vi "play-AFM-CS-imaging.vi"() -> ()   [LabVIEW 2017]
uses:
  z-axis-params.ctl
  <vilib>/userdefined/High Color/nirio_resource_hc.ctl
  controls/expMetaData.ctl
  <vilib>/Utility/file.llb/Read Delimited Spreadsheet (DBL).vi
  <vilib>/FPGAPlugInAG/cRIO-9082/niLvFpga_Open_cRIO-9082.vi
  <vilib>/rvi/interface/common/dynamic/niFpgaDynamicAddResources.vi
  <vilib>/FPGAPlugInAG/Dynamic/niLvFpga_Reset_Dynamic.vi
  <vilib>/rvi/interface/common/niFpgaWaitOnOcc.vi
  <vilib>/Utility/error.llb/Error Cluster From Error Code.vi
  <vilib>/rvi/errors/niLvFpgaAdjustHostInterfaceError.vi
  <vilib>/FPGAPlugInAG/Dynamic/niLvFpga_Run_Dynamic.vi
  <vilib>/Utility/file.llb/Write Delimited Spreadsheet (DBL).vi
  <vilib>/FPGAPlugInAG/Dynamic/niLvFpga_Close_Dynamic.vi
  <userlib>/_matio/level5/Public/Write/Append Data Element.llb/Append Data Element (Anything).vi
  <vilib>/rvi/interface/nirviOpenFPGA/nirviOpenFPGA.xnode
  FPGA Bitfiles/afmimagingcontro_FPGATargetSPARTA_cs-scanning_gCu814jKz54.lvbitx
  <vilib>/rvi/interface/nirviMethod/nirviMethod.xnode
  <vilib>/rvi/interface/nirviReadWriteControl/nirviReadWriteControl.xnode
  <vilib>/rvi/interface/nirviCloseFPGA/nirviCloseFPGA.xnode
  <vilib>/FPGAPlugInAG/Dynamic/niLvFpga_ConfigureFifo_Dynamic.vi
  <vilib>/rvi/errors/niLvFpgaMergeErrorWithErrorCode.vi
  <vilib>/rvi/interface/Simulation/niFpgaSimulationCallBeginRW.vi
  <vilib>/FPGAPlugInAG/Dynamic/niLvFpga_ReadFifo_Dynamic.vi
  NiFpgaLv.dll
  <userlib>/_matio/level5.lvlib
  <vilib>/FPGAPlugInAG/Dynamic/niLvFpga_WriteFifo_Dynamic.vi
panel:
  out "Current Case":i16
  out "state counts":u64[](array[numeric])
  out "iter":i32
  out "entity-index":i16
  out "x = 0?":bool
  out "Numeric":i32
  out "error out 2":errorcluster
  out "boolean  indicators":T1
  in  "Tab Control":T2(tab)
  in  "init Z up":sgl step=0.5
  in  "trigger-0":bool
  in  "numEntities":i16
  in  "data-root":path=path "C:/Users/arnold/Documents/labview/afm_imaging/data"
  in  "TsTicks":u32=1600
  in  "collect all":bool
  in  "collect move":bool
  in  "Ki-xy":sgl=0.005
  in  "z-axis-params":T3={"TOL"=0.3, "ramp_rate"=-5e-05, "z_u_max"=5.0, "setpoint"=0.0, "Ki"=0.01, "Z_error_threshold"=0.05, "Z_settled_samples_threshold "=500, "z_UP"=1.5, "zup_N"=500} {"Z_error_threshold" format="%#_13g"; "ramp_rate" format="%#_4g"; "TOL" format="%#_13g"}
  in  "step_down_frac":fxp<+,8,1>=1.0
  in  "input-file-name":string="cs-traj10-500.csv"
  out "output-data-path":path
  out "output-meta-data-path":path
  in  "note-blob":string
  in  "overwrite":bool
  in  "xy settled-samples\n threshold":i16=200
  in  "xy error-threshold":sgl=0.1
  out "number-settled-samples-x":i16
  out "number-settled-samples-y":i16
  out "case-selected":i16
  out "e(0) (threshhold init)":fxp<+/-,16,5>
  out "size(s)":i32
  out "nsamps":i32
  out "elements left":i32=1
  out "y iter":i32
  out "size(s) 2":i32[](array[numeric])
  out "Array":i32[][](array[numeric])
  out "z-control":dbl[](graph)
  out "x-axis":dbl[](graph)
  out "z-error":dbl[](graph)
  out "y-axis":dbl[](graph)
  in  "STOP":bool
  # "- If collect all = fasle and collect move = false,\nwe only collect measurement data.\n- If collect all = false, and collect move = true,\nwe collect measurement and move data.\n- If collect all = true, we collect everything."
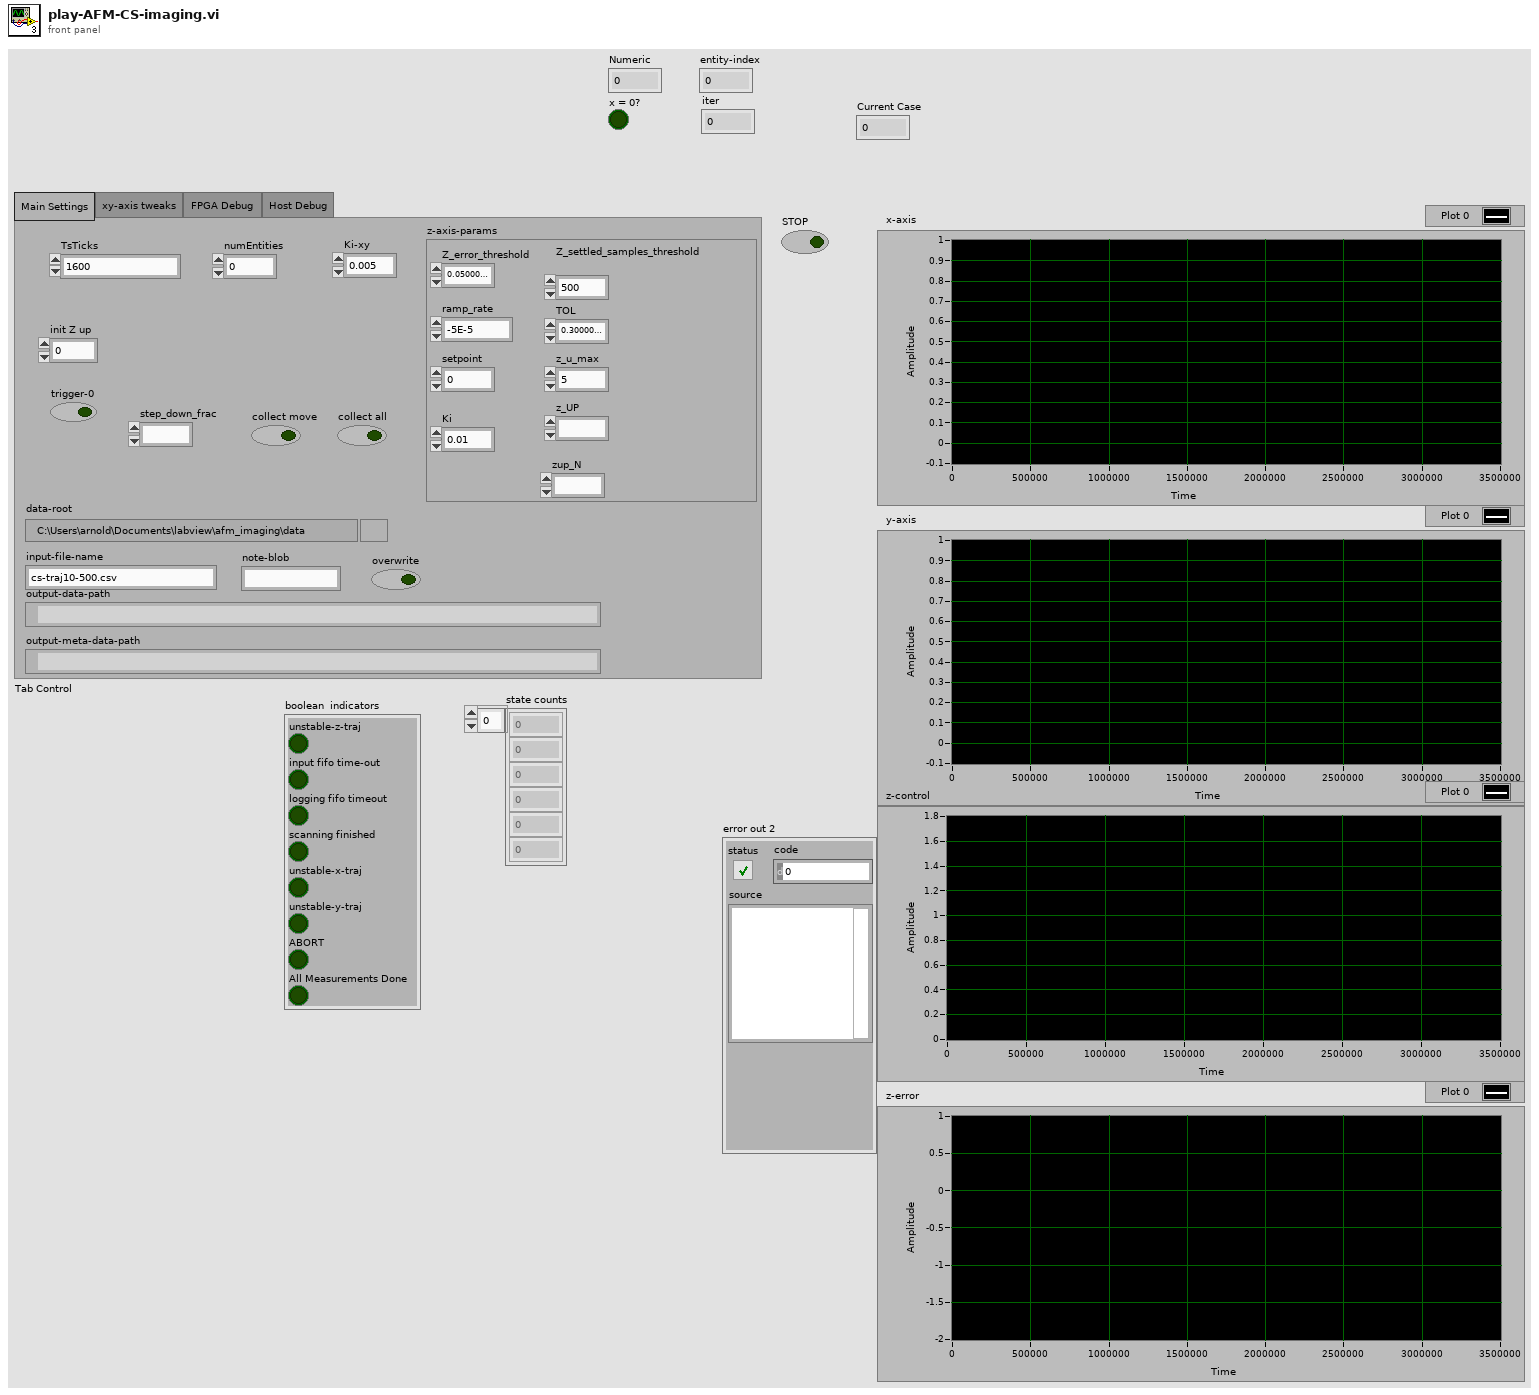
[diagram p1: front panel]
types:
  T1 = cluster{"unstable-z-traj":bool, "input fifo time-out":bool, "logging fifo timeout":bool, "scanning finished":bool, "unstable-x-traj":bool, "unstable-y-traj":bool, "ABORT":bool, "All Measurements Done":bool}
  T2 = enum32{"Main Settings", "xy-axis tweaks", "FPGA Debug ", "Host Debug"}
  T3 = typedef "z-axis-params.ctl" = cluster{"TOL":sgl, "ramp_rate":sgl, "z_u_max":sgl, "setpoint":sgl, "Ki":sgl, "Z_error_threshold":sgl, "Z_settled_samples_threshold ":i16, "z_UP":fxp<+/-,16,5>, "zup_N":i16}
  T4 = typedef "nirio_resource_hc.ctl" = tag
  T5 = enum16{"open", "replace", "create", "open or create", "replace or create", "replace or create with confirmation"}
  T6 = typedef "expMetaData.ctl" = cluster{"xy_error_threshold":sgl, "xy_settled_samples_threshold":i16, "Ki_xy":sgl, "state_counts":dbl[], "TOL":sgl, "ramp_rate":sgl, "z_u_max":sgl, "setpoint":sgl, "Ki":sgl, "Z_error_threshold":sgl, "Z_settled_samples_threshold ":i16, "z_UP":sgl, "zup_N":i16}
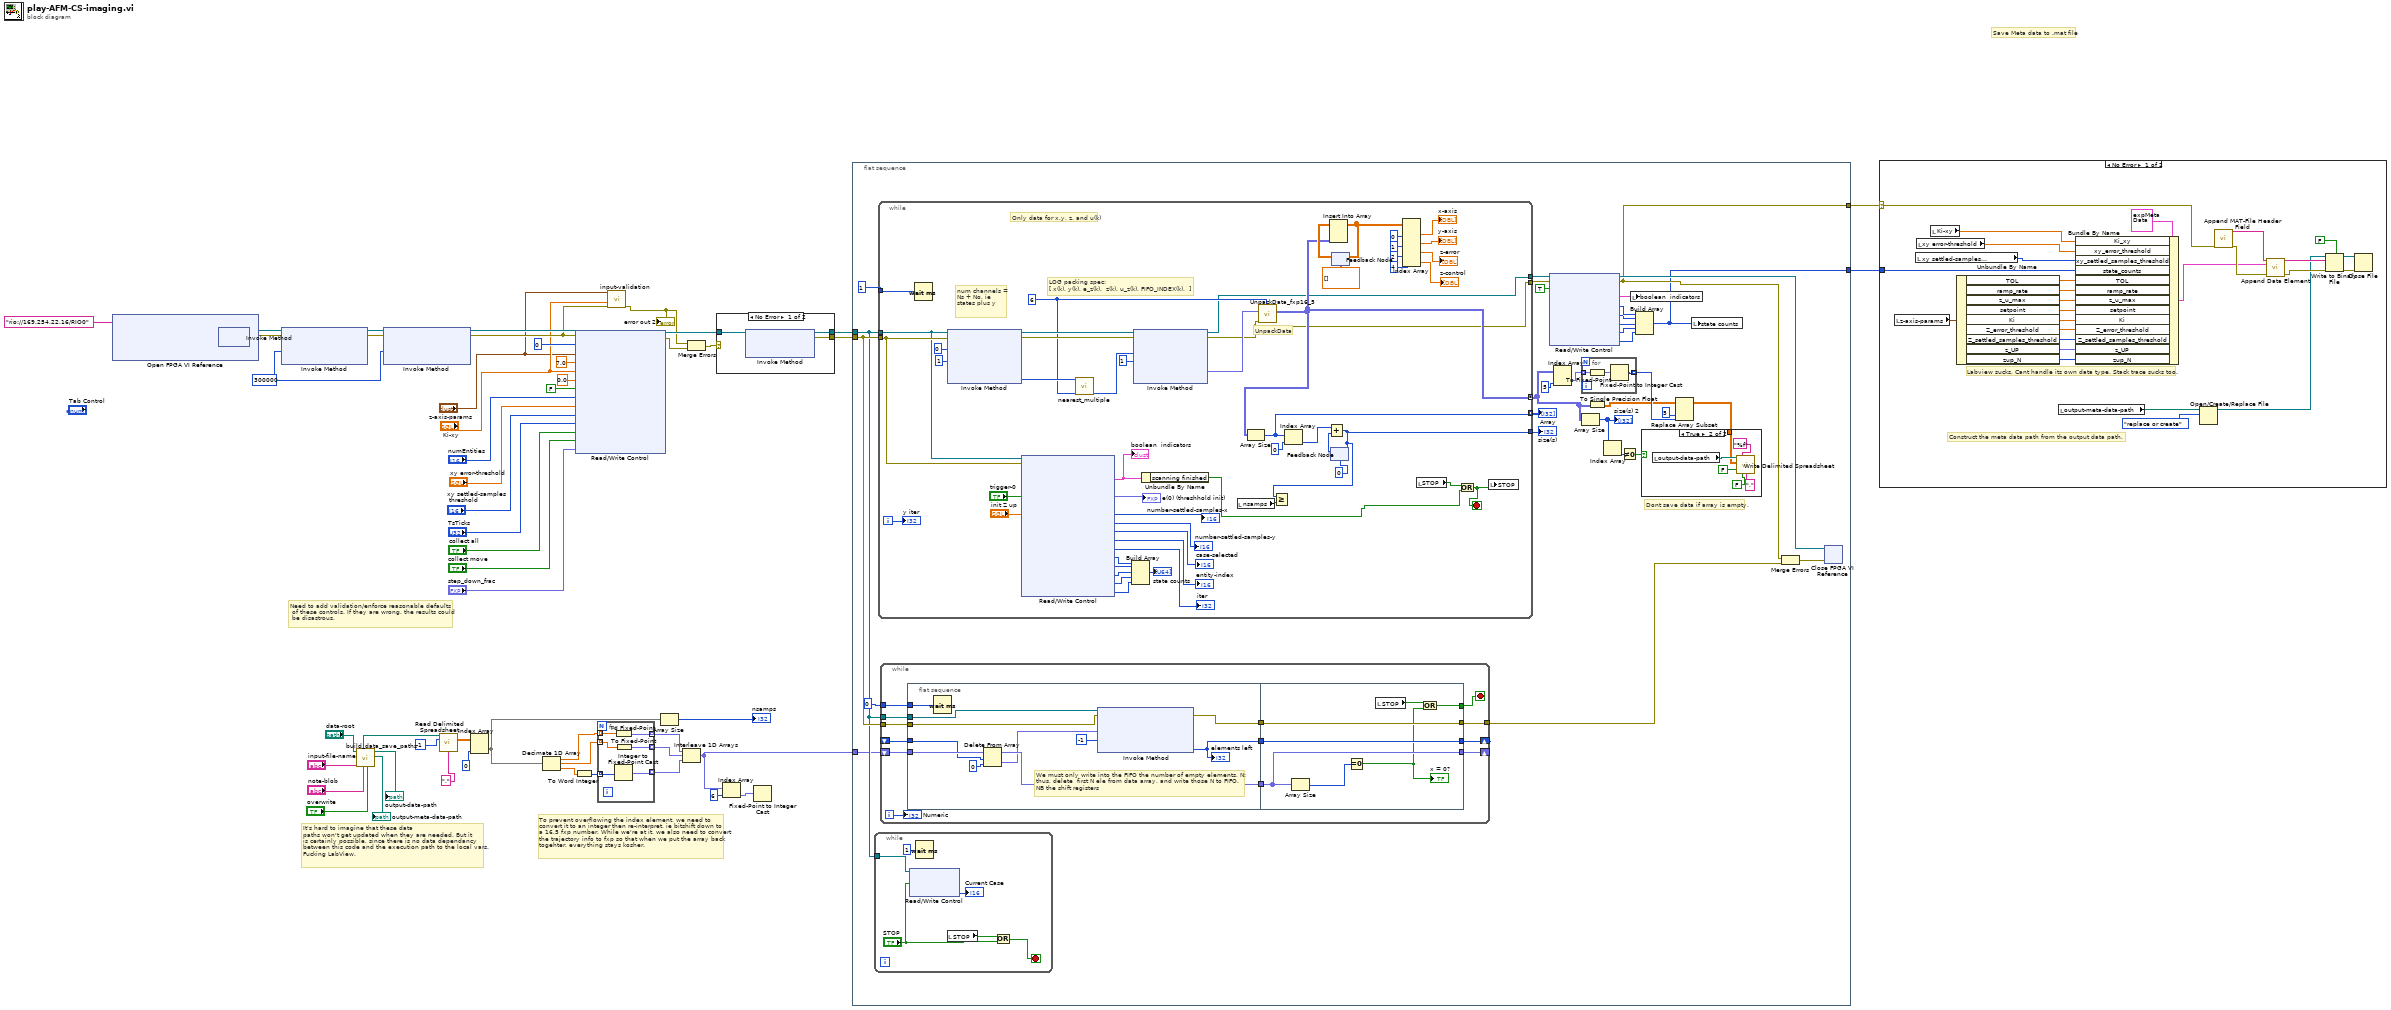
[diagram p0: block diagram]
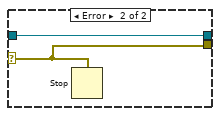
[diagram p4: hidden frame]
diagram:
  w53 = 300000
  # "It's hard to imagine that these data\npaths won't get updated when they are needed. But it \nis certainly possible, since there is no data dependancy \nbetween this code and the execution path to the local vars.\nFucking LabView."
  # "Save Meta data to .mat file"
  # "To prevent overflowing the index element, we need to \nconvert it to an integer then re-interpret, ie bitshift down to \na 16,5 fxp number. While we're at it, we also need to convert\nthe trajectory info to fxp so that when we put the array back\ntogehter, everything stays kosher."
  # "Need to add validation/enforce reasonable defaults\n of these controls. If they are wrong, the results could\n be disastrous."
  n1 = xnode "Open FPGA VI Reference"("resource name"=T4 "rio://169.254.22.16/RIO0") -> ("FPGA VI Reference Out"=w52:refnum<k20>, "error out"=w51:errorcluster)  [unwired: 1 in]
  n2 = xnode "Invoke Method"("FPGA VI Reference In"=w52, "error in"=w51) -> ("FPGA VI Reference Out"=w44:refnum<k20>, "error out"=w43:errorcluster)
  n3 = xnode "Invoke Method"("FPGA VI Reference In"=w44, "error in"=w43, "Requested Depth"=w53) -> ("FPGA VI Reference Out"=w46:refnum<k20>, "error out"=w47:errorcluster)  [unwired: 1 out]
  n4 = call "build_data_save_paths.vi"("overwrite"="overwrite", "note-blob"="note-blob", "base-file-name"="input-file-name", "data-root"="data-root") -> ("output-meta-data-path"=→"output-meta-data-path":path, "output-data-path"=→"output-data-path":path, "input-data-path"=w3:path)  [unwired: 3 in, 2 out]
  n5 = xnode "Invoke Method"("FPGA VI Reference In"=w46, "error in"=w47, "Requested Depth"=w53) -> ("FPGA VI Reference Out"=w54:refnum<k20>, "error out"=w29:errorcluster)  [unwired: 1 out]
  n6 = call-poly <vilib>:"Read Delimited Spreadsheet.vi"("file path (dialog if empty)"=w3, "number of rows (all:-1)"=-1, "delimiter (\\t)"=",") -> ("all rows"=w38:dbl[][])  [unwired: 7 in, 5 out]
  n7 = Index Array(array=w38, index (col)=0 ("dimension size")) -> (element=w14:dbl[])  [unwired: 1 in]
  n8 = Decimate 1D Array(w14) -> (w22:dbl[], w21:dbl[], w23:dbl[])
  n9 = xnode "Read/Write Control"("FPGA VI Reference In"=w54, "error in"=w29, "initial case"=i16 0, "z-axis-params"="z-axis-params", "xy-bound"=sgl 7.0, "Ki-xy"="Ki-xy", "init Z up"=sgl 0.0 ("u(0)"), "trigger-0"=FALSE, "numEntities"="numEntities", "error-threshold"="xy error-threshold", "settled-samples threshold"="xy settled-samples\n threshold", "TsTicks"="TsTicks", "collect all"="collect all", "collect move"="collect move", "step_down_frac"="step_down_frac") -> ("FPGA VI Reference Out"=w45:refnum<k20>, "error out"=w26:errorcluster)
  n10 = To Word Integer(number=w23) -> (16bit integer=w20:i16[])
  n11 = for {
    tunnel: w22 -> [w60] mode=indexing
    tunnel: w21 -> [w59] mode=indexing
    tunnel: [w58] -> w18 mode=indexing
    tunnel: [w57] -> w19 mode=indexing
    tunnel: w20 -> [w56] mode=indexing
    tunnel: [w55] -> w17 mode=indexing
    n12 = Integer to Fixed-Point Cast(integer=w56) -> (fixed-point=w55:fxp<+/-,16,5>)  [unwired: 1 in]
    n13 = To Fixed-Point(number=w60) -> (fixed-point=w57:fxp<+/-,16,5>)  [unwired: 1 in]
    n14 = To Fixed-Point(number=w59) -> (fixed-point=w58:fxp<+/-,16,5>)  [unwired: 1 in]
  }
  n15 = call "input-validation.vi"("error constant"=w29, "Ki-xy"="Ki-xy", "z-axis-params"="z-axis-params") -> ("error out"=w25:errorcluster)  [unwired: 8 in]
  "error out 2" <- w25
  n16 = Array Size(array=w14) -> (size(s)=→"nsamps":i32)
  n17 = Interleave 1D Arrays(w19, w18, w17) -> (w13:fxp<+/-,16,5>[])
  n18 = Merge Errors(w25, w26) -> (w24:errorcluster)
  n19 = case shown="No Error" w24 {
    selector: w24 -> [_ w64]
    tunnel: [w63 w64] -> w48
    tunnel: w45 -> [w62 w65]
    tunnel: [w61 w65] -> w36
    frame No Error {
      n20 = xnode "Invoke Method"("FPGA VI Reference In"=w62) -> ("FPGA VI Reference Out"=w61:refnum<k20>, "error out"=w63:errorcluster)  [unwired: 2 in]
    }
    frame Error {
      n21 = Stop(stop? (T)=w64) -> ()
    }
  }
  n22 = Index Array(array=w13, index=6) -> (element=w16:fxp<+/-,16,5>)
  n23 = Fixed-Point to Integer Cast(1:w16) -> ()  [unwired: 1 out]
  n24 = flat-sequence {
    tunnel: w48 -> [w92]
    tunnel: w36 -> [w86]
    tunnel: w13 -> [w83]
    tunnel: [w71] -> w10
    tunnel: [w70] -> w9
    frame #0 {
      # "Dont save data if array is empty."
      n25 = while {
        tunnel: w86 -> [w111]
        stop <- w107 stop-if-true
        n26 = xnode "Read/Write Control"("FPGA VI Reference In"=w111, "ABORT"="STOP") -> ("Current Case"=→"Current Case":i16)  [unwired: 1 in, 2 out]
        n27 = Wait (ms)(milliseconds to wait=u32 1) -> ()  [unwired: 1 out]
        n28 = local read "STOP"() -> (w108:bool)
        n29 = Or(x=w108, y="STOP") -> (x .or. y?=w107:bool)
      }
      n30 = while {
        tunnel: 1 -> [w194]
        tunnel: w86 -> [w182]
        tunnel: w92 -> [w183]
        tunnel: [w143] -> w90
        tunnel: [w155] -> w78 mode=concatenating
        tunnel: [w180] -> w95
        tunnel: [w153] -> w89
        tunnel: [w171] -> w85 mode=indexing
        i -> [w181]
        stop <- w172 stop-if-true
        w156 = u32 6 ("y")
        # "LOG packing spec:\n[ x(k), y(k), e_z(k),  z(k), u_z(k), FIFO_INDEX(k),  ]"
        # "num channels = Ns + No, ie states plus y"
        # "Only data for x,y, z, and u(k)"
        # "UnpackData"
        n31 = Wait (ms)(milliseconds to wait=w194) -> ()  [unwired: 1 out]
        n32 = xnode "Invoke Method"("FPGA VI Reference In"=w182, "error in"=w183, "Number of Elements"=0 ("Timeout (ms)"), "Timeout (ms)"=1) -> ("FPGA VI Reference Out"=w190:refnum<k20>, "error out"=w191:errorcluster, "Elements Remaining"=w176:u32)  [unwired: 1 out]
        n33 = xnode "Read/Write Control"("FPGA VI Reference In"=w182, "error in"=w183, "trigger-0"="trigger-0", "init Z up"="init Z up") -> ("boolean  indicators"=w174:T1, "e(0) (threshhold init)"=→"e(0) (threshhold init)":fxp<+/-,16,5>, "number-settled-samples-x"=→"number-settled-samples-x":i16, "number-settled-samples-y"=→"number-settled-samples-y":i16, "Current Case"=→"case-selected":i16, "entity-index"=→"entity-index":i16, "iter"=→"iter":i32, "state1-count"=w149:u64, "state2-count"=w148:u64, "state3-count"=w147:u64, "state4-count"=w146:u64, "state5-count"=w145:u64)  [unwired: 1 in, 2 out]
        "boolean  indicators" <- w174
        n34 = call "nearest_multiple.vi"("numChan"=w156, "N"=w176) -> ("(int) y*floor(x/y)"=w175:u64)  [unwired: 9 in]
        n35 = Build Array(w149, w148, w147, w146, w145) -> (→"state counts":u64[])
        n36 = xnode "Invoke Method"("FPGA VI Reference In"=w190, "error in"=w191, "Number of Elements"=w175, "Timeout (ms)"=1) -> ("FPGA VI Reference Out"=w143:refnum<k20>, "error out"=w153:errorcluster, "Data"=w154:fxp<+/-,16,5>[])  [unwired: 1 out]
        n37 = Unbundle By Name(w174) -> ("scanning finished"=w152:bool)
        n38 = local read "nsamps"() -> (w187:i32)
        n39 = call "UnpackData_fxp16_5.vi"("NumChannels"=w156, "error In"=w153, "1D Data In"=w154) -> ("2D Data Out"=w155:fxp<+/-,16,5>[][])  [unwired: 7 in, 1 out]
        n40 = Array Size(array=w155) -> (size(s)=w171:i32[])
        n41 = Index Array(array=w171, index=0) -> (element=w185:i32)
        n42 = feedback #1(0) -> (w186:i32)
        n43 = Add(x=w185, y=w186) -> (x+y=w180:i32)
        n44 = Greater Or Equal?(x=w180, y=w187) -> ()  [unwired: 1 out]
        n45 = feedback-in #1(w180) -> ()
        n46 = feedback #2(dbl[][] []) -> (w166:dbl[][])
        n47 = Insert Into Array(array=w166, new element=w155) -> (w157:dbl[][])  [unwired: 2 in]
        n48 = feedback-in #2(w157) -> ()
        n49 = Index Array(array=w157, index (col) #1=0 ("disabled index (col)"), index (col) #2=1 ("index (col)"), index (col) #3=2 ("index (col)"), index (col) #4=4 ("index (col)")) -> (element #1=→"x-axis":dbl[], element #2=→"y-axis":dbl[], element #3=→"z-error":dbl[], element #4=→"z-control":dbl[])  [unwired: 4 in]
        n50 = local read "STOP"() -> (w173:bool)
        n51 = Or(x=w173, y=w152) -> (x .or. y?=w172:bool)
        n52 = local write "STOP"(w172) -> ()
        "y iter" <- w181
      }
      "size(s)" <- w95
      "Array" <- w85
      n53 = while {
        tunnel: [w122] -> w91
        tunnel: 0 -> [w124]
        shift-right: [w118] -> _
        shift-left: _ -> [w121]
        shift-right: [w116] -> _
        shift-left: w83 -> [w123]
        tunnel: w86 -> [w115]
        tunnel: w92 -> [w114]
        i -> [w112]
        stop <- w113 stop-if-true
        n54 = flat-sequence {
          tunnel: w124 -> [w135]
          tunnel: w123 -> [w130]
          tunnel: w121 -> [w126]
          tunnel: [w133] -> w120
          tunnel: [w131] -> w119
          tunnel: [w132] -> w117
          tunnel: w115 -> [w128]
          tunnel: w114 -> [w127]
          tunnel: [w142] -> w118
          tunnel: [w139] -> w122
          tunnel: w120 -> [w139]
          tunnel: w119 -> [w142]
          tunnel: w117 -> [w140]
          tunnel: [w140] -> w116
          tunnel: [w136] -> w113
          frame #0 {
            # "We must only write into the FIFO the number of empty elements, N:\nthus, delete  first N ele from data array, and write those N to FIFO.\nNB the shift registers"
            n55 = Wait (ms)(milliseconds to wait=w135) -> ()  [unwired: 1 out]
            n56 = Delete From Array(array=w130, length=w126, index=0) -> (deleted portion=w129:fxp<+/-,16,5>[], array with subset deleted=w132:fxp<+/-,16,5>[])
            n57 = xnode "Invoke Method"("FPGA VI Reference In"=w128, "error in"=w127, "Data"=w129, "Timeout (ms)"=-1) -> ("error out"=w133:errorcluster, "Empty Elements Remaining"=w131:u32)  [unwired: 1 out]
            "elements left" <- w131
          }
          frame #1 {
            n58 = Array Size(array=w140) -> (size(s)=w141:i32)
            n59 = Equal To 0?(x=w141) -> (x = 0?=w138:bool)
            "x = 0?" <- w138
            n60 = local read "STOP"() -> (w137:bool)
            n61 = Or(x=w137, y=w138) -> (x .or. y?=w136:bool)
          }
        }
        "Numeric" <- w112
      }
      n62 = xnode "Read/Write Control"("FPGA VI Reference In"=w90, "error in"=w89, "ABORT"=TRUE) -> ("FPGA VI Reference Out"=w87:refnum<k20>, "error out"=w71:errorcluster, "boolean  indicators"=w84:T1, "state1-count"=w76:u64, "state2-count"=w75:u64, "state3-count"=w74:u64, "state4-count"=w73:u64, "state5-count"=w72:u64)
      n63 = Index Array(array=w78, index (col)=5) -> (element=w81:fxp<+/-,16,5>[])  [unwired: 1 in]
      n64 = for {
        tunnel: w81 -> [w104] mode=indexing
        tunnel: [w105] -> w79 mode=indexing
        n65 = To Fixed-Point(number=w104) -> (fixed-point=w103:fxp<+/-,16,5>)  [unwired: 1 in]
        n66 = Fixed-Point to Integer Cast(1:w103) -> (0:w105:i16)
      }
      n67 = Array Size(array=w78) -> (size(s)=w66:i32[])
      "size(s) 2" <- w66
      n68 = To Single Precision Float(number=w78) -> (single precision float=w77:sgl[][])
      n69 = Index Array(array=w66) -> (element=w67:i32)  [unwired: 1 in]
      n70 = Not Equal To 0?(x=w67) -> (x != 0?=w68:bool)
      n71 = local write "boolean  indicators"(w84) -> ()
      n72 = Build Array(w76, w75, w74, w73, w72) -> (w70:u64[])
      n73 = Replace Array Subset(array=w77, new element=w79, index (col)=5) -> (w69:sgl[][])  [unwired: 1 in]
      n74 = case shown="True" w68 {
        tunnel: w69 -> [_ w97]
        frame False {
        }
        frame True {
          n75 = local read "output-data-path"() -> (w102:path)
          n76 = call-poly <vilib>:"Write Delimited Spreadsheet.vi"("file path (dialog if empty)"=w102, "format (%.3f)"="%f", "2D data"=w97, "append to file? (new file:F)"=FALSE, "transpose? (no:F)"=FALSE, "delimiter (\\t)"=",") -> ()  [unwired: 8 in, 2 out]
        }
      }
      n77 = local write "state counts"(w70) -> ()
      n78 = Merge Errors(w71, w91) -> (w93:errorcluster)
      n79 = xnode "Close FPGA VI Reference"("FPGA VI Reference In"=w87, "error in"=w93) -> ()  [unwired: 1 out]
    }
  }
  n80 = case shown="No Error" w10 {
    selector: w10 -> [w214 _]
    tunnel: w9 -> [w201 _]
    frame No Error {
      # "Construct the meta data path from the output data path."
      # "Labview sucks. Cant handle its own data type. Stack trace sucks too."
      n81 = local read "z-axis-params"() -> (w200:T3)
      n82 = local read "xy settled-samples\n threshold"() -> (w197:i16)
      n83 = local read "xy error-threshold"() -> (w198:sgl)
      n84 = local read "Ki-xy"() -> (w199:sgl)
      n85 = Unbundle By Name(w200) -> ("TOL"=w211:sgl, "ramp_rate"=w210:sgl, "z_u_max"=w209:sgl, "setpoint"=w208:sgl, "Ki"=w207:sgl, "Z_error_threshold"=w206:sgl, "Z_settled_samples_threshold"=w205:i16, "z_UP"=w204:fxp<+/-,16,5>, "zup_N"=w203:i16)
      n86 = local read "output-meta-data-path"() -> (w195:path)
      n87 = Bundle By Name(cluster=T6 {"xy_error_threshold"=0.1, "xy_settled_samples_threshold"=200, "Ki_xy"=0.005, "state_counts"=[], "TOL"=0.3, "ramp_rate"=-5e-06, "z_u_max"=5.0, "setpoint"=0.0, "Ki"=0.001, "Z_error_threshold"=0.0, "Z_settled_samples_threshold "=0, "z_UP"=1.5, "zup_N"=5000} ("ExpMetaData"), "Ki_xy"=w199, "xy_error_threshold"=w198, "xy_settled_samples_threshold"=w197, "state_counts"=w201, "TOL"=w211, "ramp_rate"=w210, "z_u_max"=w209, "setpoint"=w208, "Ki"=w207, "Z_error_threshold"=w206, "Z_settled_samples_threshold"=w205, "z_UP"=w204, "zup_N"=w203) -> (w212:T6)
      n88 = Open/Create/Replace File(file path (use dialog)=w195, operation (0:open)=T5."replace or create") -> (refnum out=w213:refnum<file>)  [unwired: 4 in, 2 out]
      n89 = call <userlib>:"Append MAT-File Header Field.vi"("error"=w214) -> ("result string"=w221:string, "error out"=w215:errorcluster)  [unwired: 13 in]
      n90 = call-poly <userlib>:"Append Data Element.vi"("initial string"=w221, "data"=w212, "error in (no error)"=w215) -> ("result string"=w219:string, "error out"=w220:errorcluster)  [unwired: 11 in]
      n91 = Write to Binary File(file (use dialog)=w213, data=w219, error in=w220, 5:FALSE ("prepend array or string size? (T)")) -> (refnum out=w216:refnum<file>, error out=w217:errorcluster)  [unwired: 2 in, 1 out]
      n92 = Close File(refnum=w216, error in=w217) -> ()  [unwired: 2 out]
    }
    frame Error {
    }
  }
